vi "查询设备信息解析.vi"(9 "读取的字节":i32, 10 "响应":string) -> (1 "SN":string="FFFFFFFFFFFFFFFFFFFFFFFF", 3 "型号":string="MTM-SS2450-201")   [LabVIEW 2015]
panel:
  # "$RDEVINFO:MTM-SS2450-201,FFFFFFFFFFFFFFFFFFFFFFFF;"
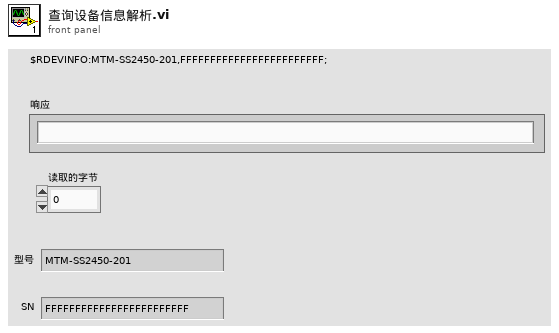
[diagram p1: front panel]
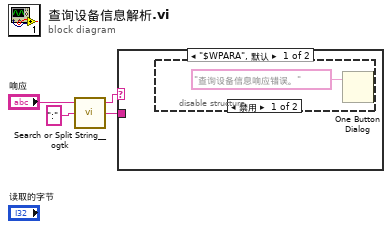
[diagram p0: block diagram]
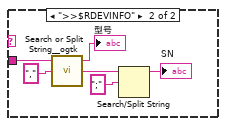
[diagram p3: hidden frame]
diagram:
  n1 = call <userlib>:"Search or Split String__ogtk.vi"("search string/char (-)"=":", "string"="响应") -> ("substring after match"=w1:string, "substring before match"=w2:string)  [unwired: 1 in, 1 out]
  n2 = case shown="\"$WPARA\", 默认" w2 {
    tunnel: w1 -> [_ w11]
    frame "$WPARA", Default {
      n3 = disable-structure shown="禁用" {
        frame Disabled {
          n4 = One Button Dialog(message="查询设备信息响应错误。" ("消息")) -> ()  [unwired: 1 in, 1 out]
        }
        frame Enabled {
        }
      }
    }
    frame ">>$RDEVINFO" {
      n5 = call <userlib>:"Search or Split String__ogtk.vi"("search string/char (-)"=",", "string"=w11) -> ("substring after match"=w8:string, "substring before match"=→"型号":string)  [unwired: 1 in, 1 out]
      n6 = Search/Split String(string=w8, search string/char (-)=";" ("搜索字符串/字符(-)")) -> (substring before match=→"SN":string)  [unwired: 1 in, 2 out]
    }
  }
